vi "Do.vi"(8 "error in (no error)":errorcluster, 10 "Actor in":refnum<class "Actor.lvclass">, 11 "QueryParameters Msg":refnum<class "QueryParameters Msg.lvclass">) -> (0 "error out":errorcluster, 2 "Actor out":refnum<class "Actor.lvclass">)   [LabVIEW 2023, in "HRS_Spectrometer.lvlib" / "QueryParameters Msg.lvclass"]
doc: "This VI delivers the message to the actor by calling the appropriate method(s) on the actor."
uses:
  QueryParameters Msg.lvclass
  QueryParameters Msg.lvclass/QueryParameters Msg.ctl
  9ef47adc-f318-494c-9b8b-6df3216d6863.vi
  HRS_Spectrometer/HRS_Spectrometer.lvclass
  <vilib>/ActorFramework/Actor/Actor.lvclass
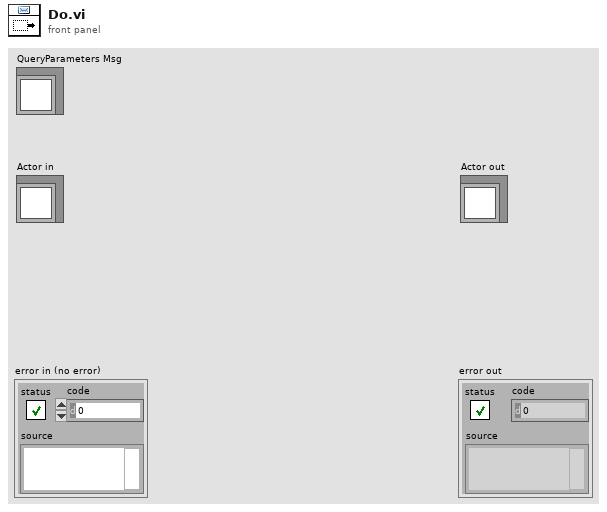
[diagram p1: front panel]
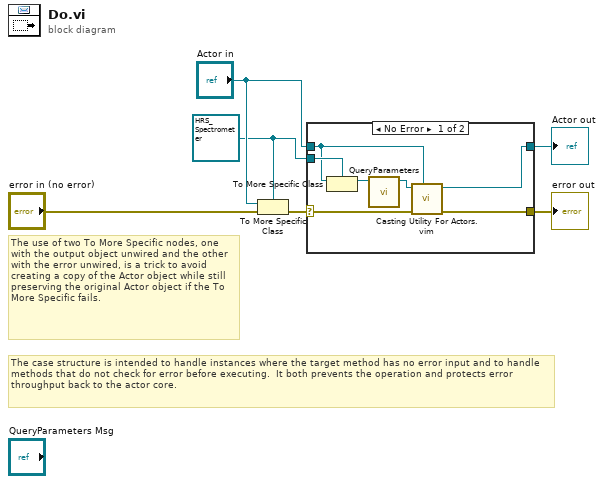
[diagram p0: block diagram]
diagram:
  w1 = refnum<class "HRS_Spectrometer.lvclass"> refnum ("Actor in")
  # "The use of two To More Specific nodes, one with the output object unwired and the other with the error unwired, is a trick to avoid creating a copy of the Actor object while still preserving the original Actor object if the To More Specific fails."
  # "The case structure is intended to handle instances where the target method has no error input and to handle methods that do not check for error before executing.  It both prevents the operation and protects error throughput back to the actor core."
  n1 = To More Specific Class(target class=w1, reference="Actor in", error in="error in (no error)") -> (error out=w5:errorcluster)  [unwired: 1 out]
  n2 = case shown="No Error" w5 {
    selector: w5 -> [w13 w15]
    tunnel: [w9 w15] -> w4
    tunnel: [w10 w14] -> w3
    tunnel: "Actor in" -> [w11 w14]
    tunnel: w1 -> [w12 _]
    frame No Error {
      n3 = To More Specific Class(target class=w12, reference=w11) -> (specific class reference=w8:refnum<class "HRS_Spectrometer.lvclass">)  [unwired: 1 in, 1 out]
      n4 = call-dynamic "QueryParameters.vi"("HRS_Spectrometer in"=w8) -> ("HRS_Spectrometer out"=w7:refnum<class "HRS_Spectrometer.lvclass">)  [unwired: 9 in, 1 out]
      n5 = call "Casting Utility For Actors.vim"("type"=w11, "error in (no error)"=w13, "Actor in"=w7) -> ("error out"=w9:errorcluster, "Actor out"=w10:refnum<class "Actor.lvclass">)  [unwired: 7 in]
    }
    frame Error {
      # "If type check fails, pass the original object out again."
    }
  }
  "error out" <- w4
  "Actor out" <- w3
